vi "SignalGenerator.vi"() -> ()   [LabVIEW 2014]
panel:
  out "error in (no error)":errorcluster
  out "error out":errorcluster
  in  "Amplitude":dbl
  in  "Frequency":dbl
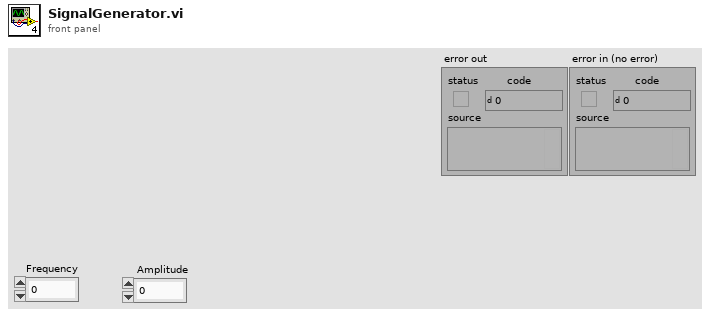
[diagram p1: front panel]
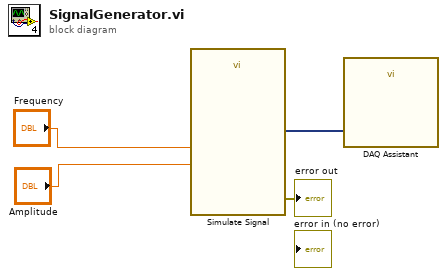
[diagram p0: block diagram]
diagram:
  n1 = call "Simulate Signal"("Frequency"="Frequency", "Amplitude"="Amplitude") -> ("Sine"=w2:dynamicdata, "error out"=→"error out":errorcluster)  [unwired: 12 in]
  n2 = call "DAQ Assistant"("data"=w2) -> ()  [unwired: 17 in, 2 out]
